vi "type_44_timestamp_three_segments.vi"   [LabVIEW 2010]
types:
  T1 = enum16{"open", "open or create", "create or replace", "create", "open (read-only)"}
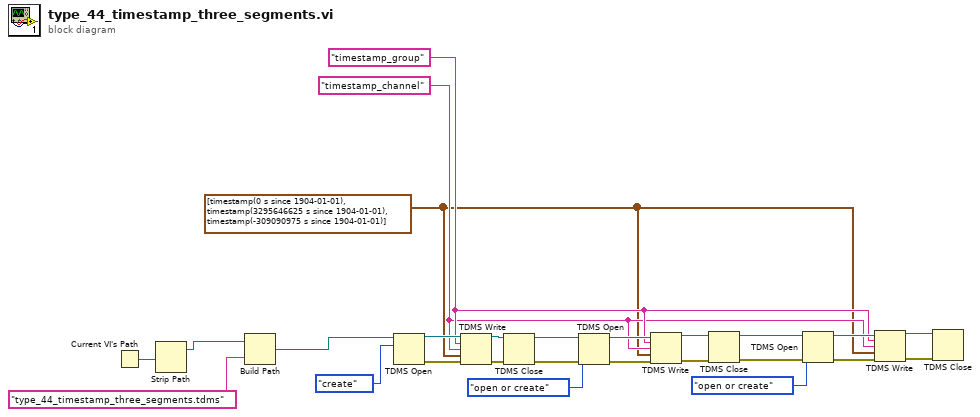
[diagram p0: block diagram]
diagram:
  w1 = timestamp[] [timestamp(0 s since 1904-01-01), timestamp(3295646625 s since 1904-01-01), timestamp(-309090975 s since 1904-01-01)]
  w2 = "timestamp_channel" ("channel name(s) in (Untitled)")
  w3 = "timestamp_group" ("group name in (Untitled)")
  n1 = Current VI's Path() -> (path=w21:path)
  n2 = Strip Path(path=w21) -> (stripped path=w20:path)  [unwired: 1 out]
  n3 = Build Path(base path=w20, name or relative path="type_44_timestamp_three_segments.tdms") -> (appended path=w18:path)
  n4 = TDMS Open(10:T1."create" ("operation (0:open)"), 11:w18) -> (0:w26:errorcluster, 3:w25:refnum<k34>)  [unwired: 4 in]
  n5 = TDMS Write(0:w25, 5:w3, 7:w2, 9:w1, 11:w26) -> (4:w23:refnum<k34>, 15:w22:errorcluster)  [unwired: 1 in, 2 out]
  n6 = TDMS Close(8:w22, 11:w23) -> (0:w15:errorcluster, 3:w17:path)
  n7 = TDMS Open(8:w15, 10:T1."open or create" ("operation (0:open)"), 11:w17) -> (0:w14:errorcluster, 3:w13:refnum<k34>)  [unwired: 3 in]
  n8 = TDMS Write(0:w13, 5:w3, 7:w2, 9:w1, 11:w14) -> (4:w11:refnum<k34>, 15:w12:errorcluster)  [unwired: 1 in, 2 out]
  n9 = TDMS Close(8:w12, 11:w11) -> (0:w4:errorcluster, 3:w5:path)
  n10 = TDMS Open(8:w4, 10:T1."open or create" ("operation (0:open)"), 11:w5) -> (0:w9:errorcluster, 3:w8:refnum<k34>)  [unwired: 3 in]
  n11 = TDMS Write(0:w8, 5:w3, 7:w2, 9:w1, 11:w9) -> (4:w6:refnum<k34>, 15:w7:errorcluster)  [unwired: 1 in, 2 out]
  n12 = TDMS Close(8:w7, 11:w6) -> ()  [unwired: 2 out]
